vi "Array 2.vi"() -> ()   [LabVIEW 2022 SP3]
panel:
  out "index of element":i32
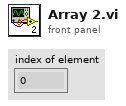
[diagram p1: front panel]
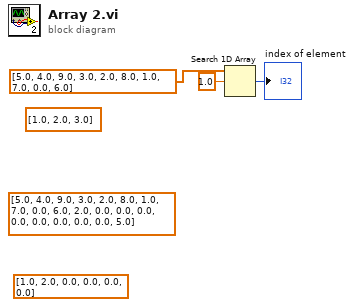
[diagram p0: block diagram]
diagram:
  (unwired) dbl[] [1.0, 2.0, 3.0]
  (unwired) dbl[] [1.0, 2.0, 0.0, 0.0, 0.0, 0.0]
  (unwired) dbl[][] [[5.0, 4.0, 9.0, 3.0, 2.0, 8.0, 1.0, 7.0, 0.0, 6.0], [2.0, 0.0, 0.0, 0.0, 0.0, 0.0, 0.0, 0.0, 0.0, 5.0]]
  n1 = Search 1D Array(1D array=dbl[] [5.0, 4.0, 9.0, 3.0, 2.0, 8.0, 1.0, 7.0, 0.0, 6.0], element=1.0) -> (index of element=→"index of element":i32)  [unwired: 1 in]
